vi "Ex14 Enhanced Object Tracking PRJ.vi"() -> ()   [LabVIEW 2020]
panel:
  out "error out":errorcluster
  out "RGB IMG":T1(plugin-control)
  out "Circles Data (calibrated)":T2(array[cluster])
  out "BINARY IMG":T1(plugin-control)
  in  "Stop (F)":bool
  # "EX.14 ENHANCED OBJECT TRACKING PRJ"
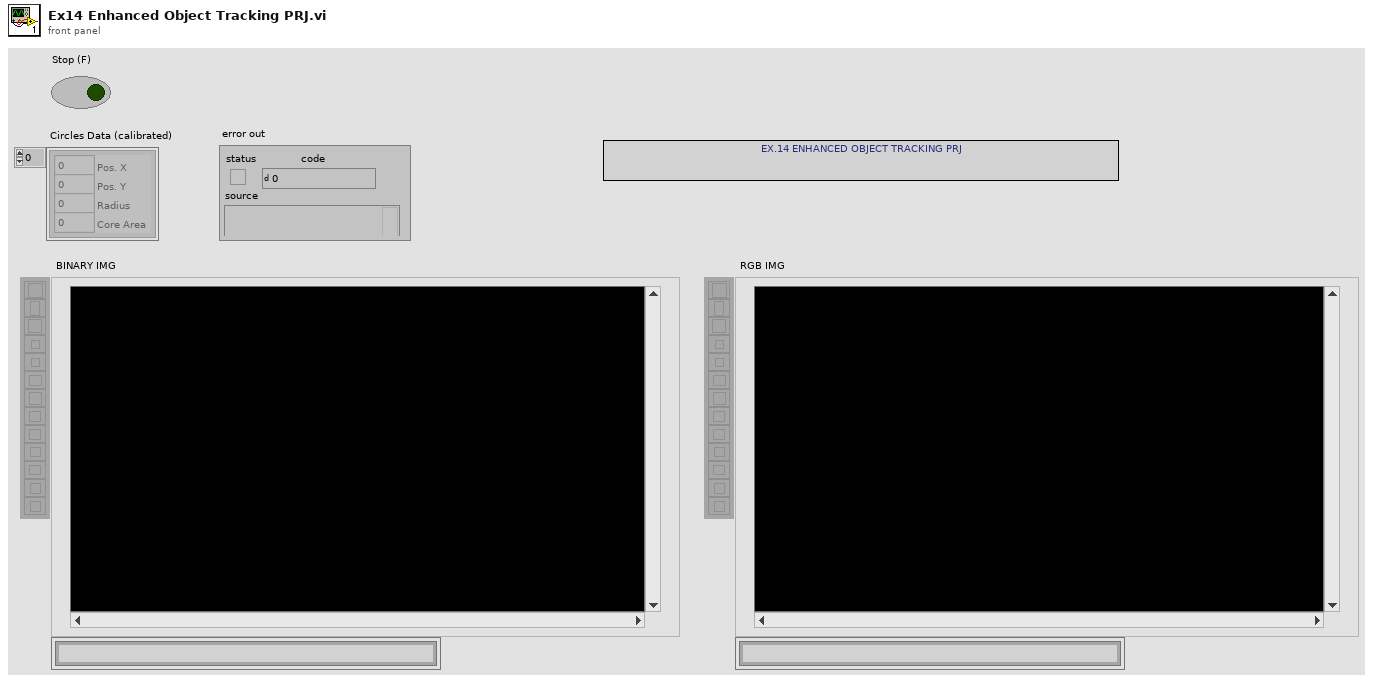
[diagram p1: front panel]
types:
  T1 = typedef "IMAQ Image.ctl" = refnum<image>
  T2 = cluster{"Pos. X":i32, "Pos. Y":i32, "Radius":i32, "Core Area":i32}[]
  T3 = cluster{"Pos. X":i32, "Pos. Y":i32, "Radius":i32, "Core Area":i32}
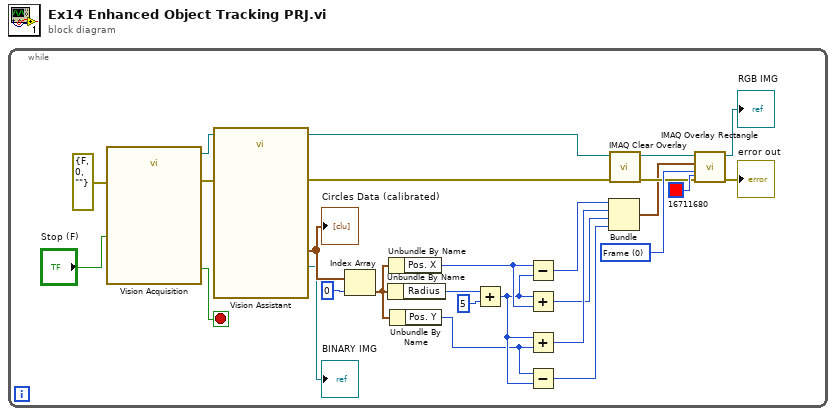
[diagram p0: block diagram]
diagram:
  n1 = while {
    stop <- w26 stop-if-true
    w13 = u32 0 items=["Frame", "Fill", "Highlight"] ("Drawing Mode (Frame)")
    n2 = call "Vision Acquisition"("Stop (F)"="Stop (F)", "error in"=errorcluster {"status"=FALSE, "code"=0, "source"=""}) -> ("Image Out"=w5:T1, "Stopped"=w26:bool, "error out"=w14:errorcluster)  [unwired: 22 in, 1 out]
    n3 = call "Vision Assistant"("Image In"=w5, "error in"=w14) -> ("Image Out"=w2:T1, "Circles Data (calibrated) (Circle Detection 1)"=w9:T2, "Image Buffer (Image Buffer 3)"=→"BINARY IMG":T1, "error out"=w7:errorcluster)  [unwired: 20 in, 2 out]
    "Circles Data (calibrated)" <- w9
    n4 = Index Array(array=w9, index=0) -> (element=w25:T3)
    n5 = Unbundle By Name(w25) -> ("Radius"=w24:i32)
    n6 = Unbundle By Name(w25) -> ("Pos. X"=w22:i32)
    n7 = Unbundle By Name(w25) -> ("Pos. Y"=w20:i32)
    n8 = Add(x=w24, y=5) -> (x+y=w21:i32)
    n9 = Subtract(x=w22, y=w21) -> (x-y=w19:i32)
    n10 = Add(x=w21, y=w22) -> (x+y=w17:i32)
    n11 = Add(x=w21, y=w20) -> (x+y=w18:i32)
    n12 = Subtract(x=w20, y=w21) -> (x-y=w16:i32)
    n13 = Bundle(w19, w18, w17, w16) -> (w1:cluster{i32, i32, i32, i32})  [unwired: 1 in]
    n14 = call "IMAQ Clear Overlay"("error in (no error)"=w7, "Image"=w2) -> ("error out"=w6:errorcluster, "Image Out"=w4:T1)  [unwired: 8 in]
    n15 = call "IMAQ Overlay Rectangle"("Color"=u32 16711680, "error in (no error)"=w6, "Drawing Mode (Frame)"=w13, "Rectangle"=w1, "Image"=w4) -> ("error out"=→"error out":errorcluster, "Image Out"=→"RGB IMG":T1)  [unwired: 5 in]
  }
